vi "RSZVB Set Alternate Sweep Mode.vi"(8 "error in (no error)":errorcluster {"code" format="%.0x"}, 9 "Alternate Sweep Mode (0: Normal)":i32(ring) items=["Normal", "Alternate"], 10 "Channel (1)":i32=1, 11 "VISA session":refnum<visa-resource-name>) -> (0 "error out":errorcluster {"code" format="%.0x"}, 3 "dup VISA session":refnum<visa-resource-name>)   [LabVIEW 2011]
doc: "This VI activates normal or alternate sweep mode.\n\nNote(s):\n\n(1) This VI is available only on R&S ZVA instrument.\n\nRemote-control command(s):\n[SENSe<Ch>:]COUPle ALL | NONE"
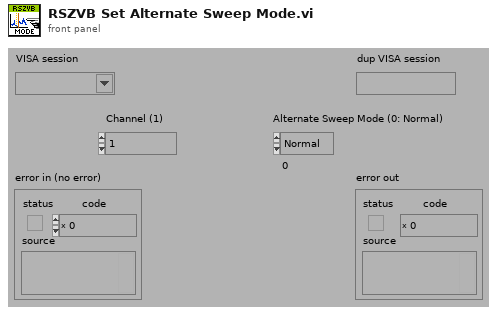
[diagram p1: front panel]
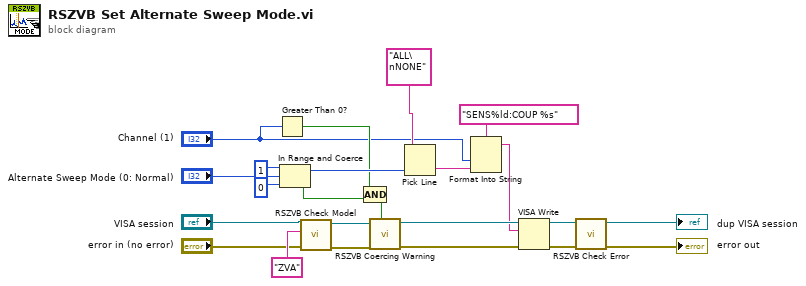
[diagram p0: block diagram]
diagram:
  n1 = Greater Than 0?(x="Channel (1)") -> (x > 0?=w12:bool)
  n2 = In Range and Coerce(upper limit=1, x="Alternate Sweep Mode (0: Normal)", lower limit=0) -> (coerced(x)=w20:i32, In Range?=w13:bool)
  n3 = call "RSZVB Check Model.vi"("error in (no error)"="error in (no error)", "Model"="ZVA" ("Options"), "VISA session"="VISA session") -> ("error out"=w1:errorcluster, "dup VISA session"=w2:refnum<visa-resource-name>)  [unwired: 7 in]
  n4 = Compound Arithmetic op=AND(w12, w13) -> (w11:bool)
  n5 = call "RSZVB Coercing Warning.vi"("In Range?"=w11, "error in (no error)"=w1, "VISA session"=w2) -> ("error out"=w17:errorcluster, "dup VISA session"=w18:refnum<visa-resource-name>)  [unwired: 7 in]
  n6 = Pick Line(multi-line string="ALL\nNONE", line index=w20) -> (output string=w14:string)  [unwired: 1 in]
  n7 = Format Into String(format string="SENS%ld:COUP %s", "Channel (1)", w14) -> (resulting string=w10:string)  [unwired: 2 in, 1 out]
  n8 = VISA Write(VISA resource name=w18, write buffer=w10, error in (no error)=w17) -> (VISA resource name out=w15:refnum<visa-resource-name>, error out=w16:errorcluster)  [unwired: 1 out]
  n9 = call "RSZVB Check Error.vi"("error in (no error)"=w16, "VISA session"=w15) -> ("error out"=→"error out":errorcluster, "dup VISA session"=→"dup VISA session":refnum<visa-resource-name>)  [unwired: 8 in]
